vi "MGCC_StaEst_initial_input.vi"   [LabVIEW 2016]
types:
  T1 = cluster{"V_node":cdb[][], "P_node":cdb[][], "I_node":cdb[][], "NumN":dbl, "NumL":dbl, "Ybus":cdb[][], "sspn":dbl[][], "ssqn":dbl[][], "ssvn":dbl[][], "SlackBus":dbl, "Topology":dbl[][]}
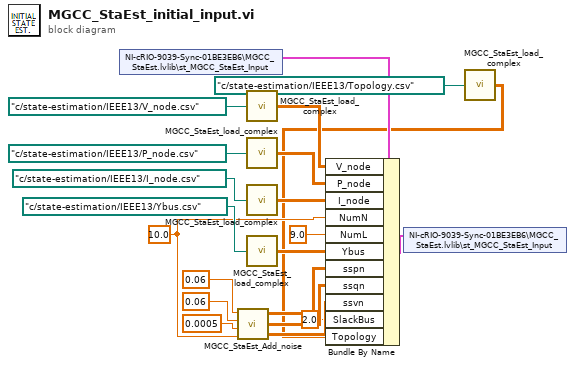
[diagram p0: block diagram]
diagram:
  w4 = 10.0 ("NumN")
  n1 = shared-variable "NI-cRIO-9039-Sync-01BE3EB6\\MGCC_StaEst.lvlib\\st_MGCC_StaEst_Input"() -> (w20:T1)  [unwired: 1 in, 1 out]
  n2 = call "MGCC_StaEst_Add_noise.vi"("Node"=w4, "svn"=0.0005, "sqn"=0.06, "spn"=0.06) -> ("ssvn"=w10:dbl[][], "ssqn"=w11:dbl[][], "sspn"=w12:dbl[][])
  n3 = call "MGCC_StaEst_load_complex.vi"("file path (dialog if empty)"=path "c:/state-estimation/IEEE13/V_node.csv" ("file path (use dialog)")) -> ("Array 13"=w16:cdb[][])
  n4 = call "MGCC_StaEst_load_complex.vi"("file path (dialog if empty)"=path "c:/state-estimation/IEEE13/P_node.csv" ("file path (use dialog)")) -> ("Array 13"=w8:cdb[][])
  n5 = call "MGCC_StaEst_load_complex.vi"("file path (dialog if empty)"=path "c:/state-estimation/IEEE13/I_node.csv" ("file path (use dialog)")) -> ("Array 13"=w18:cdb[][])
  n6 = call "MGCC_StaEst_load_complex.vi"("file path (dialog if empty)"=path "c:/state-estimation/IEEE13/Ybus.csv" ("file path (use dialog)")) -> ("Array 13"=w5:cdb[][])
  n7 = call "MGCC_StaEst_load_complex.vi"("file path (dialog if empty)"=path "c:/state-estimation/IEEE13/Topology.csv" ("file path (use dialog)")) -> ("Array 13"=w1:cdb[][])
  n8 = Bundle By Name(cluster=w20, "V_node"=w16, "P_node"=w8, "I_node"=w18, "NumN"=w4, "NumL"=9.0, "Ybus"=w5, "sspn"=w12, "ssqn"=w11, "ssvn"=w10, "SlackBus"=2.0, "Topology"=w1) -> (w21:T1)
  n9 = shared-variable "NI-cRIO-9039-Sync-01BE3EB6\\MGCC_StaEst.lvlib\\st_MGCC_StaEst_Input"(w21) -> ()  [unwired: 1 in, 1 out]
